vi "sendMessage.vi"(8 "error in (no error)":errorcluster, 10 "message":string, 11 "TCPClient in":refnum<class "TCPCommunication.lvclass">) -> (0 "error out":errorcluster, 3 "TCPClient out":refnum<class "TCPCommunication.lvclass">)   [LabVIEW 2016, in "TCPCommunication.lvclass"]
uses:
  TCPCommunication.lvclass
  TCPCommunication.lvclass/TCPCommunication.ctl
  common_ascii_tcp/TCPClient/TCPClient.lvclass
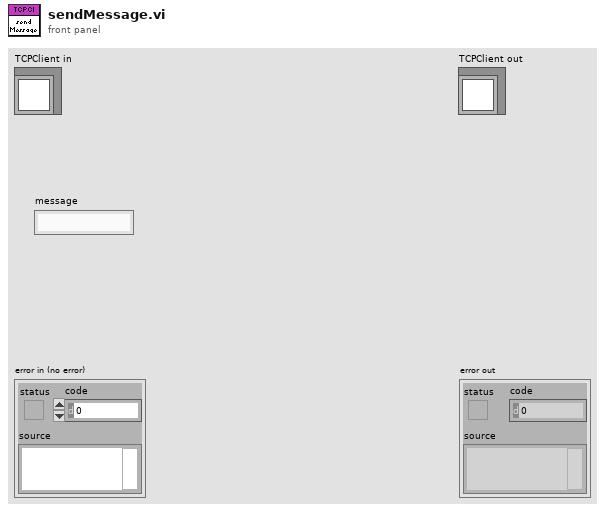
[diagram p1: front panel]
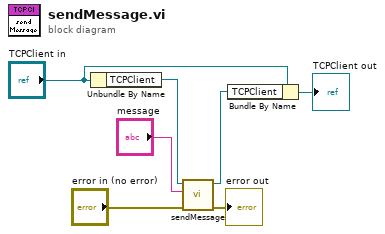
[diagram p0: block diagram]
diagram:
  n1 = Unbundle By Name("TCPClient in") -> ("TCPClient"=w5:refnum<class "TCPClient.lvclass">)
  n2 = call-dynamic "sendMessage.vi"("error in (no error)"="error in (no error)", "message"="message", "TCPClient in"=w5) -> ("error out"=→"error out":errorcluster, "TCPClient out"=w4:refnum<class "TCPClient.lvclass">)  [unwired: 7 in]
  n3 = Bundle By Name(cluster="TCPClient in", "TCPClient"=w4) -> (→"TCPClient out":refnum<class "TCPCommunication.lvclass">)
